vi "final_usrp_test.vi"() -> ()   [LabVIEW 2014]
uses:
  <vilib>/addons/Modulation/Analog/support/mod_Set Error Source.vi
  var_stop.vi
  <vilib>/addons/Modulation/Digital/Support/Common/Validators/mod_Generate Filter Coefficients Validate.vi
  <vilib>/addons/Modulation/Digital/General/subVIs/mod_Generate Filter Coefficients.vi
  <vilib>/measure/maspectr.llb/FFT Power Spectrum and PSD for 1 Chan (CDB).vi
  <vilib>/addons/Modulation/Digital/General/MT Apply Matched Filter (Generic).vi
  <vilib>/addons/Modulation/Digital/General/MT Align to Ideal Symbols (Generic).vi
  <instrlib>/niUSRP/niUSRP Fetch Rx Data (CDB Cluster).vi
  <instrlib>/niUSRP/niUSRP Write Tx Data (CDB Cluster).vi
  <vilib>/addons/Modulation/Digital/General/MT Apply Pulse Shaping Filter (Generic).vi
  <vilib>/addons/Modulation/niDMT.lvlib
  <vilib>/measure/NI_MAPro.lvlib
panel:
  out "energy detector  size":i32
  in  "frame buffer size":i32=20
  in  "Stop":bool
  out "Frames Per Second":u32
  in  "energy threshold":dbl=-33.0 format="%#_13g"
  out "elements in frame buffer 2":i32
  out "elements in frame buffer":i32
  out "valid frames":i32
  out "elements in send buffer":i32
  in  "packet size":i32=12800
  in  "Quality (0-1000)":i32=100 caption="Quality (750)"
  out "size(s) 4":i32
  out "frame num":u32
  out "length":i32[](array[numeric])
  out "start index":i32[](array[numeric])
  out "Numeric":i32
  out "size(s) 3":i32
  out "# elements in queue 2":i32
  out "size(s) 2":i32
  out "size(s)":i32[](array[numeric])
  out "image":T1(plugin-control)
  in  "Transmit power (db)":dbl
  out "found?":bool
  out "# elements in queue":i32
  out "valid?":bool
  in  "Gray code?":bool=TRUE
  in  "Modulation":enum16{"PSK", "QAM"}(ring)
  out "packet len":u32
  in  "filter length (symbols)":i32=8
  in  "filter parameter":dbl=0.5 format="%.2f"
  in  "pulse shaping filter (none)":T2(ring)=enum."Raised Cosine"
  in  "M-PSK (4)":i32=4 caption="M-ARY"
  in  "samples per symbol (16)":i32=4
  out "packet bits length":i32
  in  "number of samples":i64=40000
  out "RX coerced gain":dbl format="%#_6f"
  out "RX coerced carrier frequency":dbl=915000000.0 format="%#_6p"
  out "RX coerced IQ rate":dbl=4000000.0 format="%#_6p"
  in  "RX active antenna":string="RX2"
  in  "RX gain":dbl format="%#_6f"
  in  "RX device names":refnum<k15>="192.168.10.2"
  out "TX coerced gain":dbl format="%#_6f"
  out "TX coerced carrier frequency":dbl=915000000.0 format="%#_6p"
  out "coerced IQ rate":dbl=4000000.0 format="%#_6p"
  in  "TX device names":refnum<k15>="192.168.10.2"
  in  "TX gain":dbl format="%#_6f"
  in  "carrier frequency":dbl=915000000.0 format="%#_6p"
  in  "IQ rate":dbl=800000.0 format="%#_6p"
  in  "stop":bool
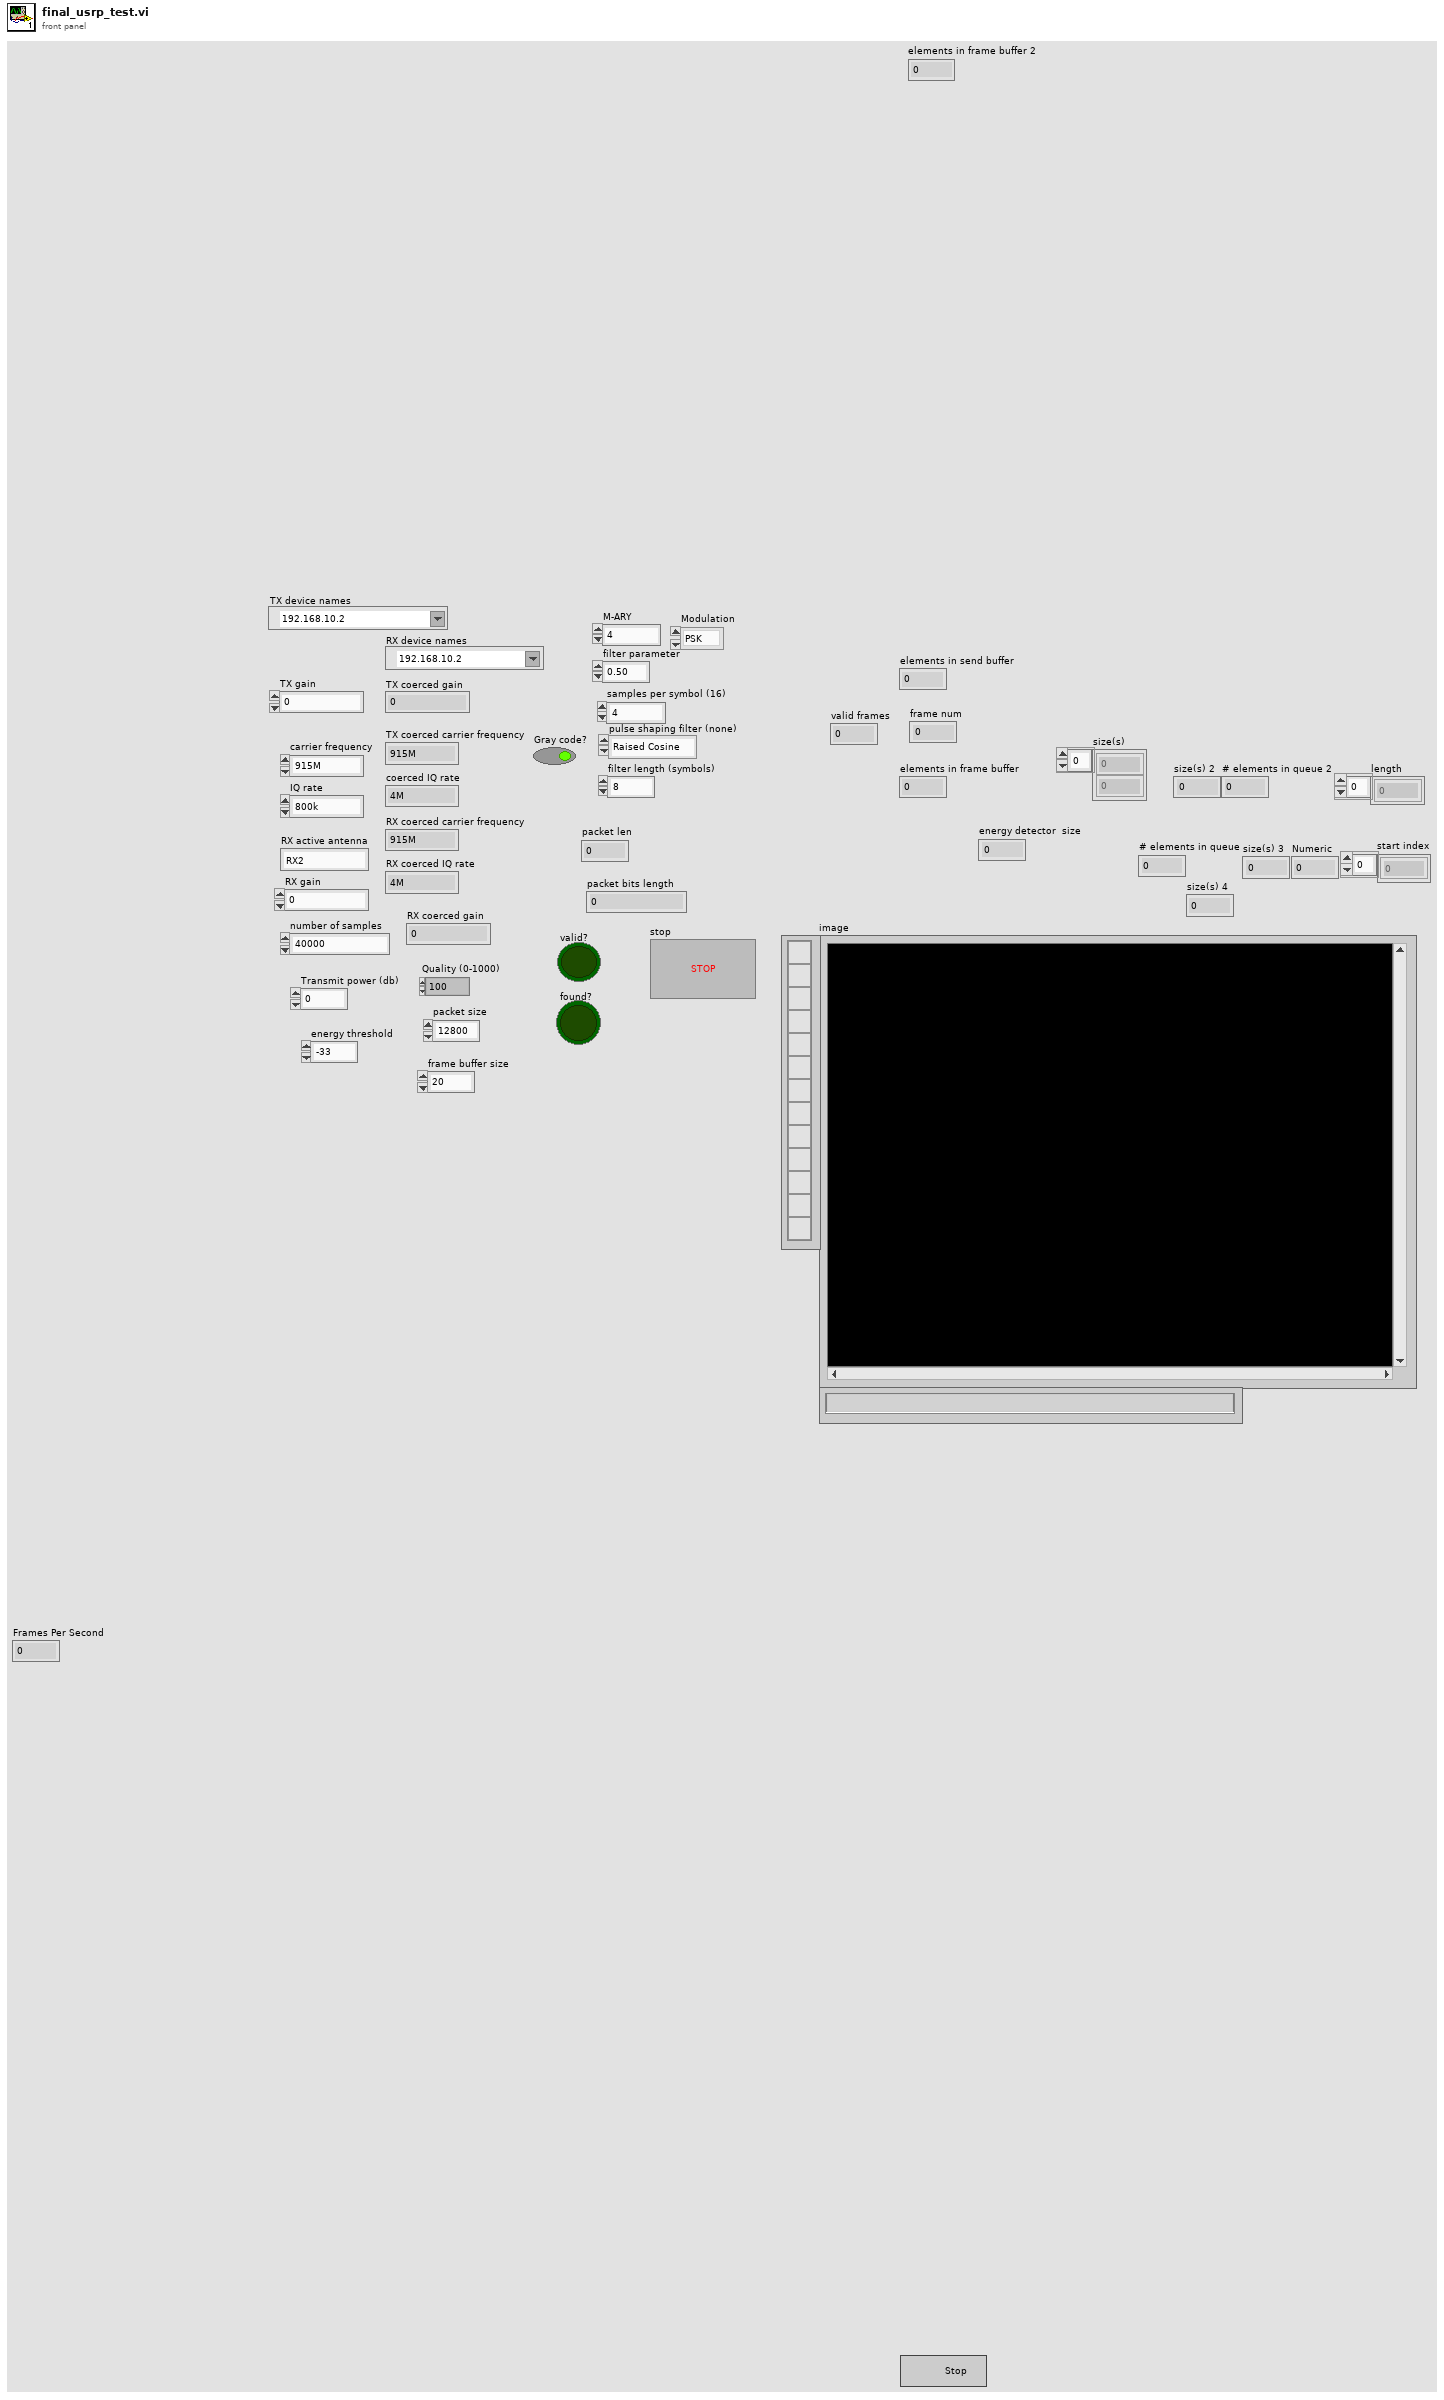
[diagram p1: front panel]
types:
  T1 = typedef "IMAQ Image.ctl" = refnum<image>
  T2 = enum16{"none", "Raised Cosine", "Root Raised Cos", "Gaussian"}
  T3 = enum16{"FSK", "PSK", "QAM", "MSK", "PAM", "ASK", "CPM"}
  T4 = cluster{"samples per symbol (16)":i32, "symbol map":cdb[], "index map":u32[]}
  T5 = cluster{"samples per symbol (16)":i32, "symbol map":cdb[], i32[]}
  T6 = typedef "IMAQ AVI2 Refnum.ctl" = refnum<k20>
  T7 = typedef "Image Type" = u32
  T8 = cluster{"Width":u32, "Height":u32, "Frames Per Second":u32, "Codec":string, "Has Data":bool}
  T9 = typedef "niAMT.lvlib/Complex Data Waveform.ctl" = cluster{"t0":dbl, "dt":dbl, "Y":cdb[]}
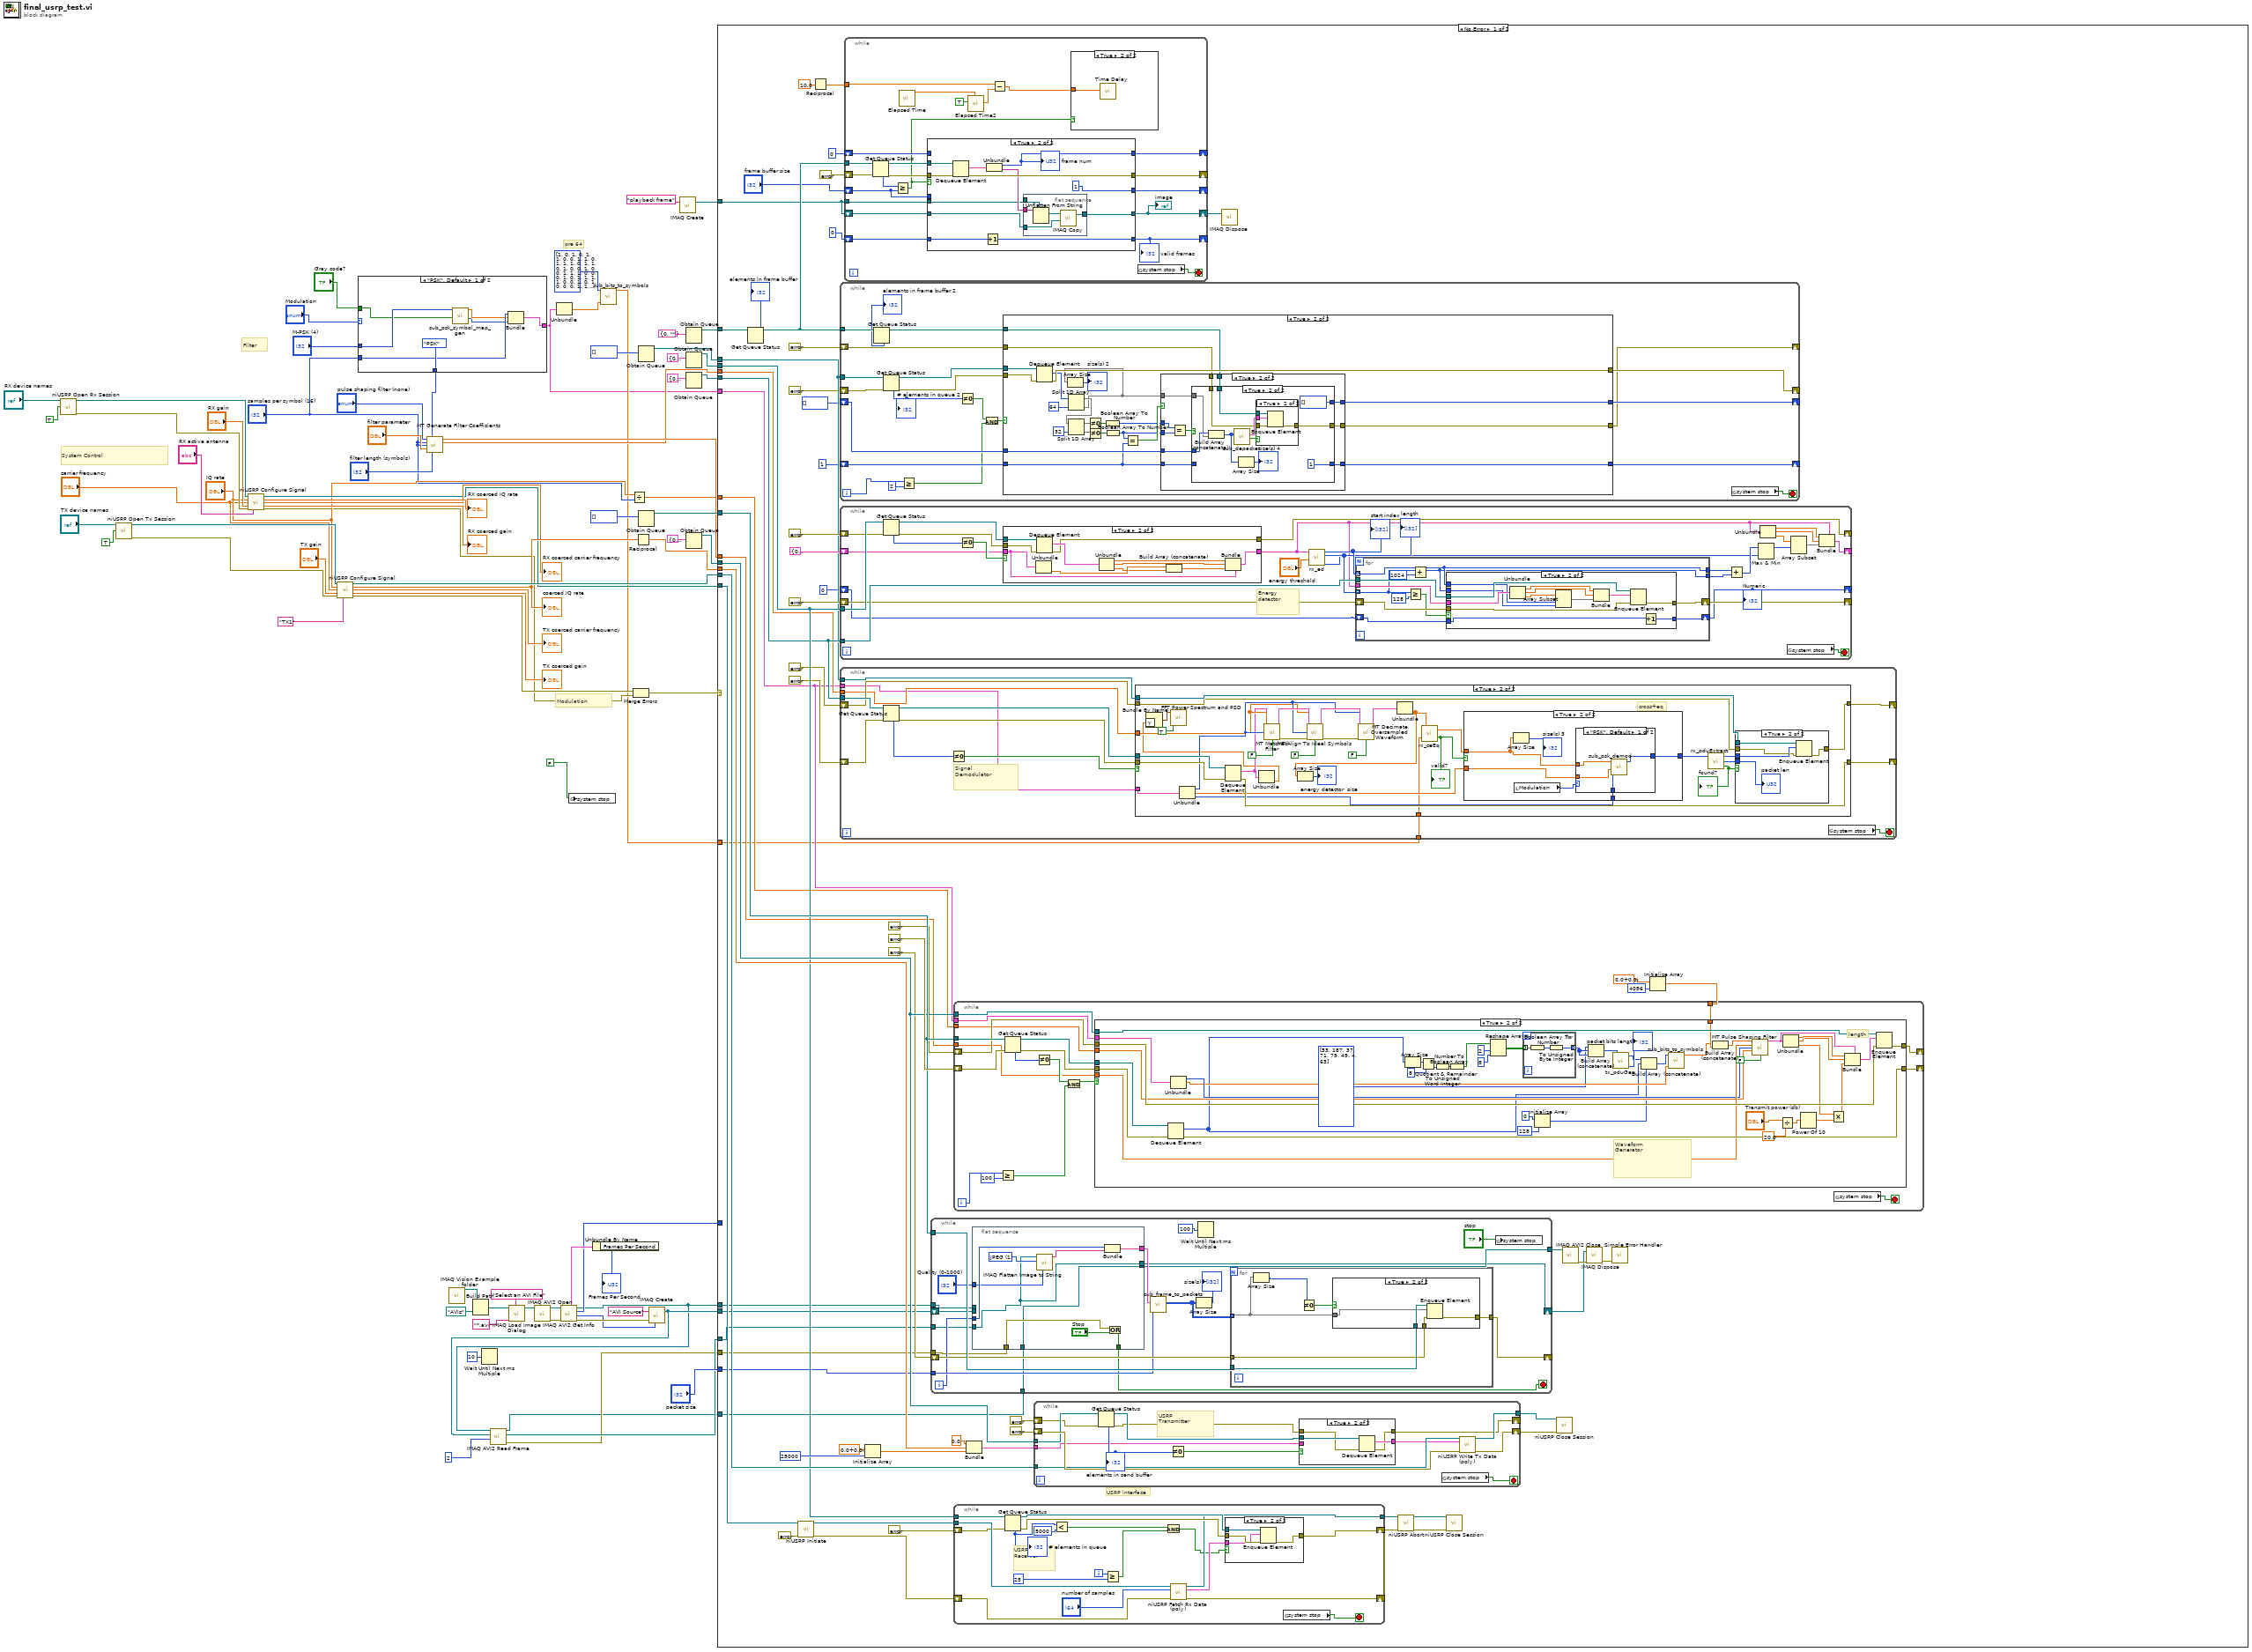
[diagram p0: block diagram]
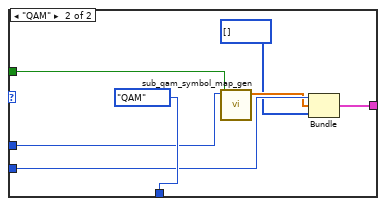
[diagram p2: hidden frame]
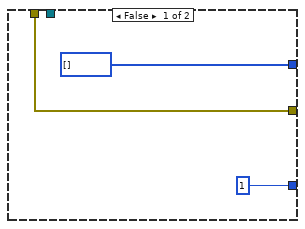
[diagram p7: hidden frame]
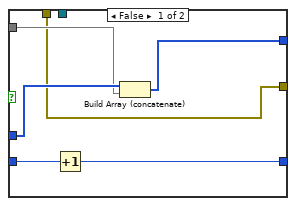
[diagram p8: hidden frame]
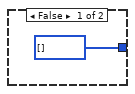
[diagram p11: hidden frame]
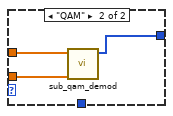
[diagram p12: hidden frame]
diagram:
  # "pre 64"
  # "Modulation"
  # "Filter"
  # "System Control"
  n1 = call <instrlib>:"niUSRP Open Rx Session.vi"("device names"="RX device names", "reset"=TRUE) -> ("session handle out"=w64:refnum<k15>, "error out"=w63:errorcluster)  [unwired: 12 in]
  n2 = call <instrlib>:"niUSRP Open Tx Session.vi"("device names"="TX device names", "reset"=TRUE) -> ("session handle out"=w77:refnum<k15>, "error out"=w76:errorcluster)  [unwired: 12 in]
  n3 = call <instrlib>:"niUSRP Configure Signal.vi"("session handle"=w64, "IQ rate"="IQ rate", "carrier frequency"="carrier frequency", "gain"="RX gain", "error in (no error)"=w63, "active antenna"="RX active antenna") -> ("session handle out"=w55:refnum<k15>, "coerced IQ rate"=→"RX coerced IQ rate":dbl, "coerced carrier frequency"=→"RX coerced carrier frequency":dbl, "coerced gain"=→"RX coerced gain":dbl, "error out"=w39:errorcluster)  [unwired: 5 in]
  n4 = call <instrlib>:"niUSRP Configure Signal.vi"("session handle"=w77, "IQ rate"="IQ rate", "carrier frequency"="carrier frequency", "gain"="TX gain", "error in (no error)"=w76, "active antenna"="TX1") -> ("session handle out"=w68:refnum<k15>, "coerced IQ rate"=w66:dbl, "coerced carrier frequency"=→"TX coerced carrier frequency":dbl, "coerced gain"=→"TX coerced gain":dbl, "error out"=w40:errorcluster)  [unwired: 5 in]
  "coerced IQ rate" <- w66
  n5 = case shown="\"PSK\", Default" "Modulation" {
    tunnel: [T3."PSK" ("modulation type") T3."QAM" ("modulation type")] -> w34
    tunnel: "M-PSK (4)" -> [w84 w90]
    tunnel: "Gray code?" -> [w83 w91]
    tunnel: "samples per symbol (16)" -> [w82 w89]
    tunnel: [w79 w86] -> w27
    frame "PSK", Default {
      n6 = call "sub_psk_symbol_map_gen.vi"("Gray code?"=w83, "M-PSK"=w84) -> ("index map"=w80:u32[], "symbol map"=w81:cdb[])  [unwired: 8 in]
      n7 = Bundle("samples per symbol (16)"=w82, "symbol map"=w81, "index map"=w80) -> (w79:T4)  [unwired: 1 in]
    }
    frame "QAM" {
      n8 = call "sub_qam_symbol_map_gen.vi"("Gray code?"=w91, "M-QAM"=w90) -> ("symbol map"=w88:cdb[])  [unwired: 9 in]
      n9 = Bundle("samples per symbol (16)"=w89, "symbol map"=w88, i32[] []) -> (w86:T5)  [unwired: 1 in]
    }
  }
  n10 = call <vilib>:"MT Generate Filter Coefficients.vi"("pulse shaping filter (none)"="pulse shaping filter (none)", "modulation type"=w34, "pulse shaping samples per symbol (16)"="samples per symbol (16)", "matched samples per symbol (16)"="samples per symbol (16)", "filter parameter"="filter parameter", "filter length (symbols)"="filter length (symbols)") -> ("pulse shaping filter coefficients"=w45:dbl[], "matched filter coefficients"=w43:dbl[])  [unwired: 7 in, 1 out]
  n11 = call "IMAQ Vision Example folder.vi"() -> ("Example Image Path"=w17:path)  [unwired: 11 in]
  n12 = Build Path(base path=w17, name or relative path=path "AVIs") -> (appended path=w14:path)
  n13 = Wait Until Next ms Multiple(millisecond multiple=u32 10) -> ()  [unwired: 1 out]
  n14 = call "IMAQ Load Image Dialog"("Prompt"="Select an AVI File" ("prompt"), "Pattern"="*.avi", "Start Path"=w14) -> ("Path"=w13:path)  [unwired: 6 in, 2 out]
  n15 = call "IMAQ AVI2 Open"("AVI File Path"=w13) -> ("error out"=w21:errorcluster, "AVI Refnum"=w20:T6)  [unwired: 2 in, 7 out]
  n16 = Unbundle(w27) -> ("symbol map"=w29:cdb[])  [unwired: 2 out]
  n17 = call "IMAQ AVI2 Get Info"("error in (no error)"=w21, "AVI Refnum"=w20) -> ("error out"=w19:errorcluster, "Image Type"=w18:T7, "Number of Frames"=w10:u32, "AVI Refnum (duplicate)"=w5:T6, "Frame Data"=w22:T8)  [unwired: 5 out]
  n18 = global write "var_stop.vi" "system stop"(FALSE) -> ()
  n19 = Unbundle By Name(w22) -> ("Frames Per Second"=→"Frames Per Second":u32)
  n20 = call "sub_bits_to_symbols.vi"("symbol map"=w29, "bits"=i16[] [1, 0, 1, 0, 1, 1, 0, 0, 1, 1, 0, 1, 1, 1, 0, 1, 1, 0, 1, 0, 0, 1, 0, 0, 1, 1, 1, 0, 0, 0, 1, 0, 1, 1, 1, 1, 0, 0, 1, 0, 1, 0, 0, 0, 1, 1, 0, 0, 0, 0, 1, 0, 0, 0, 0, 0, 1, 1, 1, 1, 1, 1, 0, 0] ("preamble(64) 2")) -> ("symbols"=w28:cdb[])  [unwired: 9 in]
  n21 = Divide(x="IQ rate", y="samples per symbol (16)") -> (x/y=w44:dbl)
  n22 = Merge Errors(w40, w39) -> (w38:errorcluster)
  n23 = Reciprocal(x=w66) -> (1/x=w65:dbl)
  n24 = Obtain Queue(element data type=i8[] [] ("output bit stream")) -> (queue out=w50:refnum<queue>)  [unwired: 4 in, 2 out]
  n25 = Obtain Queue(element data type=i16[] []) -> (queue out=w78:refnum<queue>)  [unwired: 4 in, 2 out]
  n26 = call "IMAQ Create"("Image Name"="AVI Source", "Image Type"=w18, "error in (no error)"=w19) -> ("New Image"=w6:T1)  [unwired: 1 in, 2 out]
  n27 = call "IMAQ AVI2 Read Frame"("Frame Number"=u32 2, "Image"=w6, "AVI Refnum"=w5) -> ("error out"=w2:errorcluster, "Image Out"=w3:T1, "AVI Refnum (duplicate)"=w1:T6)  [unwired: 1 in, 5 out]
  n28 = call "IMAQ Create"("Image Name"="playback frame") -> ("New Image"=w8:T1)  [unwired: 3 in, 2 out]
  n29 = Obtain Queue(element data type=cluster{u32, "string":string} {0, "string"=""} ("frame")) -> (queue out=w25:refnum<queue>)  [unwired: 4 in, 2 out]
  n30 = Obtain Queue(element data type=cluster{"t0":dbl, "dt":dbl, "Y":cdb[]} {"t0"=0.0, "dt"=0.0, "Y"=[]} ("data")) -> (queue out=w54:refnum<queue>)  [unwired: 4 in, 2 out]
  n31 = Obtain Queue(element data type=cluster{"t0":dbl, "dt":dbl, "Y":cdb[]} {"t0"=0.0, "dt"=0.0, "Y"=[]} ("data")) -> (queue out=w51:refnum<queue>)  [unwired: 4 in, 2 out]
  n32 = Obtain Queue(element data type=cluster{"t0":dbl, "dt":dbl, "Y":cdb[]} {"t0"=0.0, "dt"=1.0, "Y"=[]} ("data")) -> (queue out=w69:refnum<queue>)  [unwired: 4 in, 2 out]
  n33 = case shown="No Error" w38 {
    tunnel: w78 -> [w158 _]
    tunnel: w69 -> [w153 _]
    tunnel: w68 -> [w154 _]
    tunnel: w65 -> [w147 _]
    tunnel: w55 -> [w142 _]
    tunnel: w54 -> [w136 _]
    tunnel: w51 -> [w132 _]
    tunnel: w50 -> [w130 _]
    tunnel: w27 -> [w124 _]
    tunnel: w45 -> [w127 _]
    tunnel: w44 -> [w126 _]
    tunnel: w43 -> [w125 _]
    tunnel: w28 -> [w118 _]
    tunnel: w25 -> [w114 _]
    tunnel: "packet size" -> [w108 _]
    tunnel: w10 -> [_ _]
    tunnel: w5 -> [w103 _]
    tunnel: w6 -> [w102 _]
    tunnel: w8 -> [w96 _]
    tunnel: w3 -> [w95 _]
    tunnel: w2 -> [w94 _]
    tunnel: w1 -> [w93 _]
    frame No Error {
      # "USRP interface"
      n34 = Get Queue Status(queue=w114) -> (queue out=w106:refnum<queue>, # elements in queue=→"elements in frame buffer":i32)  [unwired: 2 in, 6 out]
      n35 = call <instrlib>:"niUSRP Initiate.vi"("session handle"=w142, "error in (no error)"=errorcluster {"status"=FALSE, "code"=0, "source"=""}) -> ("session handle out"=w141:refnum<k15>, "error out"=w140:errorcluster)  [unwired: 12 in]
      n36 = Reciprocal(x=10.0) -> (1/x=w109:dbl)
      n37 = while {
        tunnel: w130 -> [w265]
        shift-right: [w258] -> _
        shift-left: errorcluster {"status"=FALSE, "code"=0, "source"=""} ("error out") -> [w264]
        shift-right: [w256] -> _
        shift-left: u32 1 -> [w257]
        shift-right: [w255] -> _
        shift-left: i8[] [] ("second subarray") -> [w254]
        tunnel: w106 -> [w253]
        shift-right: [w251] -> _
        shift-left: errorcluster {"status"=FALSE, "code"=0, "source"=""} ("error out") -> [w252]
        i -> [w249]
        stop <- w263 stop-if-true
        n38 = Get Queue Status(queue=w253) -> (queue out=w246:refnum<queue>, # elements in queue=→"elements in frame buffer 2":i32)  [unwired: 2 in, 6 out]
        n39 = Get Queue Status(queue=w265, error in (no error)=w264) -> (queue out=w260:refnum<queue>, error out=w259:errorcluster, # elements in queue=w262:i32)  [unwired: 1 in, 5 out]
        "# elements in queue 2" <- w262
        n40 = Greater Or Equal?(x=w249, y=2) -> (x >= y?=w248:bool)
        n41 = Not Equal To 0?(x=w262) -> (x != 0?=w261:bool)
        n42 = And(x=w261, y=w248) -> (x .and. y?=w247:bool)
        n43 = case shown="True" w247 {
          tunnel: w260 -> [_ w292]
          tunnel: w259 -> [w269 w291]
          tunnel: [w269 w290] -> w258
          tunnel: w257 -> [w268 w276]
          tunnel: [w268 w277] -> w256
          tunnel: [w266 w281] -> w255
          tunnel: w254 -> [w266 w278]
          tunnel: w246 -> [_ w275]
          tunnel: w252 -> [w267 w274]
          tunnel: [w267 w273] -> w251
          frame False {
          }
          frame True {
            n44 = Dequeue Element(queue=w292, error in (no error)=w291) -> (element=w272:i8[], error out=w290:errorcluster)  [unwired: 1 in, 2 out]
            n45 = Split 1D Array(array=w272, index=64) -> (first subarray=w283:i8[], second subarray=w270:i8[])
            n46 = Array Size(array=w270) -> (size(s)=→"size(s) 2":i32)
            n47 = Split 1D Array(array=w283, index=32) -> (first subarray=w286:i8[], second subarray=w287:i8[])
            n48 = Not Equal To 0?(x=w286) -> (x != 0?=w285:bool[])
            n49 = Not Equal To 0?(x=w287) -> (x != 0?=w284:bool[])
            n50 = Boolean Array To Number(Boolean array=w285) -> (number=w280:u32)
            n51 = Boolean Array To Number(Boolean array=w284) -> (number=w279:u32)
            n52 = Equal?(x=w279, y=w276) -> (x = y?=w282:bool)
            n53 = case shown="True" w282 {
              tunnel: [i8[] [] ("second subarray") w303] -> w281
              tunnel: w280 -> [_ w306]
              tunnel: w279 -> [_ w305]
              tunnel: w278 -> [_ w302]
              tunnel: w270 -> [_ w301]
              tunnel: [u32 1 w300] -> w277
              tunnel: w276 -> [_ w299]
              tunnel: w275 -> [_ w298]
              tunnel: w274 -> [w293 w297]
              tunnel: [w293 w296] -> w273
              frame False {
              }
              frame True {
                n54 = Equal?(x=w306, y=w305) -> (x = y?=w304:bool)
                n55 = case shown="True" w304 {
                  tunnel: [w310 i8[] [] ("second subarray")] -> w303
                  tunnel: w302 -> [w312 w321]
                  tunnel: w301 -> [w311 w320]
                  tunnel: [w308 u32 1] -> w300
                  tunnel: w299 -> [w309 _]
                  tunnel: w298 -> [_ w319]
                  tunnel: w297 -> [w307 w317]
                  tunnel: [w307 w316] -> w296
                  frame False {
                    n56 = Increment(x=w309) -> (x+1=w308:u32)
                    n57 = Build Array (concatenate)(w312, w311) -> (w310:i8[])
                  }
                  frame True {
                    n58 = Build Array (concatenate)(w321, w320) -> (w315:i8[])
                    n59 = call "sub_depacket.vi"("bitstream"=w315) -> ("CRC valid"=w313:bool, "frame"=w318:cluster{u32, "string":string})  [unwired: 9 in]
                    n60 = Array Size(array=w315) -> (size(s)=→"size(s) 4":i32)
                    n61 = case shown="True" w313 {
                      tunnel: w319 -> [_ w328]
                      tunnel: w318 -> [_ w327]
                      tunnel: w317 -> [w324 w326]
                      tunnel: [w324 w325] -> w316
                      frame False {
                      }
                      frame True {
                        n62 = Enqueue Element(queue=w328, element=w327, error in (no error)=w326) -> (error out=w325:errorcluster)  [unwired: 1 in, 2 out]
                      }
                    }
                  }
                }
              }
            }
          }
        }
        n63 = global read "var_stop.vi" "system stop"() -> (w263:bool)
      }
      n64 = while {
        tunnel: w136 -> [w424]
        shift-right: [w417] -> _
        shift-left: errorcluster {"status"=FALSE, "code"=0, "source"=""} ("error out") -> [w423]
        shift-right: [w403] -> _
        shift-left: cluster{"t0":dbl, "dt":dbl, "Y":cdb[]} {"t0"=0.0, "dt"=0.0, "Y"=[]} ("data") -> [w418]
        tunnel: w132 -> [w416]
        shift-right: [w415] -> _
        shift-left: errorcluster {"status"=FALSE, "code"=0, "source"=""} ("error out") -> [w414]
        shift-right: [w398] -> _
        shift-left: 0 -> [w399]
        stop <- w413 stop-if-true
        # "Energy\ndetector"
        n65 = Get Queue Status(queue=w424, error in (no error)=w423) -> (queue out=w419:refnum<queue>, error out=w420:errorcluster, # elements in queue=w422:i32)  [unwired: 1 in, 5 out]
        n66 = Not Equal To 0?(x=w422) -> (x != 0?=w421:bool)
        n67 = case shown="True" w421 {
          tunnel: w420 -> [w453 w464]
          tunnel: w419 -> [_ w463]
          tunnel: w418 -> [w452 w458]
          tunnel: [w453 w455] -> w417
          tunnel: [w452 w454] -> w410
          frame False {
          }
          frame True {
            n68 = Unbundle(w458) -> ("Y"=w461:cdb[])  [unwired: 2 out]
            n69 = Dequeue Element(queue=w463, error in (no error)=w464) -> (element=w462:cluster{"t0":dbl, "dt":dbl, "Y":cdb[]}, error out=w455:errorcluster)  [unwired: 1 in, 2 out]
            n70 = Unbundle(w462) -> ("t0"=w457:dbl, "dt"=w456:dbl, "Y"=w460:cdb[])
            n71 = Build Array (concatenate)(w461, w460) -> (w459:cdb[])
            n72 = Bundle(cluster=w458, "t0"=w457, "dt"=w456, "Y"=w459) -> (w454:cluster{"t0":dbl, "dt":dbl, "Y":cdb[]})
          }
        }
        n73 = call "rx_ed.vi"("energy threshold"="energy threshold", "Wavefrom"=w410) -> ("first pulse"=w400:i32, "length"=w411:i32[], "start index"=w412:i32[])  [unwired: 7 in]
        "start index" <- w412
        "length" <- w411
        n74 = for {
          tunnel: w416 -> [w436]
          tunnel: w410 -> [w433]
          shift-right: [w435] -> w415
          shift-left: w414 -> [w434]
          tunnel: w412 -> [w432] mode=indexing
          tunnel: w411 -> [w431] mode=indexing
          tunnel: [w432] -> w406
          tunnel: [w426] -> w405
          shift-right: [w427] -> w398
          shift-left: w399 -> [w428]
          n75 = Greater Or Equal?(x=w431, y=128) -> (x >= y?=w429:bool)
          n76 = Add(x=w431, y=1024) -> (x+y=w426:i32)
          n77 = case shown="True" w429 {
            tunnel: w436 -> [_ w451]
            tunnel: [w438 w450] -> w435
            tunnel: w434 -> [w438 w449]
            tunnel: w433 -> [_ w448]
            tunnel: w432 -> [_ w442]
            tunnel: w426 -> [_ w441]
            tunnel: w428 -> [w437 w440]
            tunnel: [w437 w439] -> w427
            frame False {
            }
            frame True {
              n78 = Unbundle(w448) -> ("t0"=w446:dbl, "dt"=w447:dbl, "Y"=w444:cdb[])
              n79 = Array Subset(array=w444, index=w442, length=w441) -> (w443:cdb[])
              n80 = Bundle("t0"=w446, "dt"=w447, w443) -> (w445:cluster{"t0":dbl, "dt":dbl, cdb[]})  [unwired: 1 in]
              n81 = Enqueue Element(queue=w451, element=w445, error in (no error)=w449) -> (error out=w450:errorcluster)  [unwired: 1 in, 2 out]
              n82 = Increment(x=w440) -> (x+1=w439:i32)
            }
          }
        }
        "Numeric" <- w398
        n83 = Add(x=w406, y=w405) -> (x+y=w402:i32)
        n84 = Max & Min(x=w402, y=w400) -> (max(x,y)=w401:i32)  [unwired: 1 out]
        n85 = Unbundle(w410) -> ("t0"=w409:dbl, "dt"=w408:dbl, "Y"=w407:cdb[])
        n86 = global read "var_stop.vi" "system stop"() -> (w413:bool)
        n87 = Array Subset(array=w407, index=w401) -> (w404:cdb[])  [unwired: 1 in]
        n88 = Bundle(cluster=w410, "t0"=w409, "dt"=w408, "Y"=w404) -> (w403:cluster{"t0":dbl, "dt":dbl, "Y":cdb[]})
      }
      n89 = while {
        tunnel: w132 -> [w342]
        shift-right: [w336] -> _
        shift-left: errorcluster {"status"=FALSE, "code"=0, "source"=""} ("error out") -> [w341]
        tunnel: w130 -> [w335]
        shift-right: [w334] -> _
        shift-left: errorcluster {"status"=FALSE, "code"=0, "source"=""} ("error out") -> [w333]
        tunnel: w125 -> [w331]
        tunnel: w124 -> [w330]
        tunnel: w118 -> [w329]
        stop <- w332 stop-if-true
        # "Signal \nDemodulator"
        n90 = Get Queue Status(queue=w342, error in (no error)=w341) -> (queue out=w338:refnum<queue>, error out=w337:errorcluster, # elements in queue=w340:i32)  [unwired: 1 in, 5 out]
        n91 = Not Equal To 0?(x=w340) -> (x != 0?=w339:bool)
        n92 = case shown="True" w339 {
          tunnel: w338 -> [_ w375]
          tunnel: w337 -> [w344 w376]
          tunnel: [w344 w374] -> w336
          tunnel: w335 -> [_ w365]
          tunnel: [w343 w364] -> w334
          tunnel: w333 -> [w343 w363]
          tunnel: w331 -> [_ w352]
          tunnel: w330 -> [_ w356]
          tunnel: w329 -> [_ w349]
          frame False {
          }
          frame True {
            # "cross+eq"
            n93 = Unbundle(w356) -> ("samples per symbol (16)"=w355:i32, "symbol map"=w354:cdb[], "index map"=w353:u32[])
            n94 = Dequeue Element(queue=w375, error in (no error)=w376) -> (element=w348:cluster{"t0":dbl, "dt":dbl, "Y":cdb[]}, error out=w374:errorcluster)  [unwired: 1 in, 2 out]
            n95 = Unbundle(w348) -> ("Y"=w347:cdb[])  [unwired: 2 out]
            n96 = Bundle By Name("Y"=w347) -> (w351:waveform(cdb))  [unwired: 1 in]
            n97 = call-poly <vilib>:"FFT Power Spectrum and PSD.vi"("dB On (F)"=TRUE, "time signal"=w351) -> ()  [unwired: 6 in, 4 out]
            n98 = call-poly <vilib>:"MT Matched Filter.vi"("input complex waveform"=w348, "matched filter coefficients"=w352, "samples per symbol (16)"=w355, "reset? (T)"=FALSE) -> ("output complex waveform"=w373:T9, "error out"=w372:errorcluster)  [unwired: 10 in]
            n99 = call-poly <vilib>:"MT Align To Ideal Symbols.vi"("input complex waveform"=w373, "matched filter coefficients"=w352, "samples per symbol (16)"=w355, "error in (no error)"=w372, "reset? (T)"=FALSE) -> ("output complex waveform"=w370:T9, "error out"=w371:errorcluster)  [unwired: 8 in, 1 out]
            n100 = call <vilib>:"MT Decimate Oversampled Waveform.vi"("input complex waveform"=w370, "decimation factor"=w355, "error in (no error)"=w371, "reset? (T)"=FALSE) -> ("output complex waveform"=w369:T9)  [unwired: 10 in, 1 out]
            n101 = Unbundle(w369) -> ("Y"=w345:cdb[])  [unwired: 2 out]
            n102 = Array Size(array=w345) -> (size(s)=→"energy detector  size":i32)
            n103 = call "rx_ceEq.vi"("preamble"=w349, "symbols"=w345) -> ("valid?"=w361:bool, "eq symbols"=w362:cdb[])
            "valid?" <- w361
            n104 = case shown="True" w361 {
              tunnel: [i8[] [] ("output bit stream") w381] -> w368
              tunnel: w354 -> [_ w382]
              tunnel: w362 -> [_ w379]
              tunnel: w353 -> [_ w380]
              frame False {
              }
              frame True {
                n105 = Array Size(array=w379) -> (size(s)=→"size(s) 3":i32)
                n106 = local read "Modulation"() -> (w383:enum16{"PSK", "QAM"})
                n107 = case shown="\"PSK\", Default" w383 {
                  tunnel: w379 -> [w387 w390]
                  tunnel: w382 -> [w386 w389]
                  tunnel: [w384 w388] -> w381
                  tunnel: w380 -> [w385 _]
                  frame "PSK", Default {
                    n108 = call "sub_psk_demod.vi"("index map"=w385, "symbol map"=w386, "symbol"=w387) -> ("bitstream"=w384:i16[])  [unwired: 8 in]
                  }
                  frame "QAM" {
                    n109 = call "sub_qam_demod.vi"("symbol map"=w389, "symbol"=w390) -> ("bitstream"=w388:i16[])  [unwired: 9 in]
                  }
                }
              }
            }
            n110 = call "rx_pduExtract.vi"("output bit stream"=w368) -> ("found?"=w367:bool, "packet len"=w360:u32, "ppdu"=w366:i8[])  [unwired: 2 in]
            "found?" <- w367
            n111 = case shown="True" w367 {
              tunnel: w366 -> [_ w394]
              tunnel: w365 -> [_ w396]
              tunnel: [w391 w395] -> w364
              tunnel: w363 -> [w391 w392]
              tunnel: w360 -> [_ w393]
              frame False {
              }
              frame True {
                n112 = Enqueue Element(queue=w396, element=w394, error in (no error)=w392) -> (error out=w395:errorcluster)  [unwired: 1 in, 2 out]
                "packet len" <- w393
              }
            }
          }
        }
        n113 = global read "var_stop.vi" "system stop"() -> (w332:bool)
      }
      n114 = while {
        tunnel: w106 -> [w221]
        shift-right: [w217] -> _
        shift-left: errorcluster {"status"=FALSE, "code"=0, "source"=""} ("error out") -> [w220]
        shift-right: [w214] -> _
        shift-left: 0 -> [w213]
        tunnel: w109 -> [w209]
        shift-right: [w210] -> _
        shift-left: 0 -> [w211]
        shift-right: [w205] -> _
        shift-left: "frame buffer size" -> [w204]
        shift-right: [w201] -> w97
        shift-left: w96 -> [w202]
        tunnel: w96 -> [w200]
        stop <- w216 stop-if-true
        n115 = Get Queue Status(queue=w221, error in (no error)=w220) -> (queue out=w219:refnum<queue>, error out=w218:errorcluster, # elements in queue=w206:i32)  [unwired: 1 in, 5 out]
        n116 = Greater Or Equal?(x=w206, y=w204) -> (x >= y?=w203:bool)
        n117 = call "Elapsed Time"() -> ("Present (s)"=w208:dbl)  [unwired: 12 in, 7 out]
        n118 = case shown="True" w203 {
          tunnel: w219 -> [_ w239]
          tunnel: w218 -> [w227 w238]
          tunnel: [w227 w236] -> w217
          tunnel: [w226 w234] -> w214
          tunnel: w213 -> [w226 _]
          tunnel: w211 -> [w225 w233]
          tunnel: [w225 w232] -> w210
          tunnel: [w224 1] -> w205
          tunnel: w204 -> [w224 _]
          tunnel: [w223 w229] -> w201
          tunnel: w202 -> [w223 w228]
          tunnel: w200 -> [_ w230]
          frame False {
          }
          frame True {
            n119 = Dequeue Element(queue=w239, error in (no error)=w238) -> (element=w237:cluster{u32, "string":string}, error out=w236:errorcluster)  [unwired: 1 in, 2 out]
            n120 = Increment(x=w233) -> (x+1=w232:i32)
            n121 = Unbundle(w237) -> (w234:u32, "string"=w235:string)
            "frame num" <- w234
            n122 = flat-sequence {
              tunnel: w235 -> [w244]
              tunnel: w230 -> [w243]
              tunnel: [w241] -> w229
              tunnel: w228 -> [w240]
              frame #0 {
                n123 = Unflatten From String(type=w243, binary string=w244) -> (value=w242:T1)  [unwired: 3 in, 2 out]
                n124 = call "IMAQ Copy"("Image Dst"=w240, "Image Src"=w242) -> ("Image Dst Out"=w241:T1)  [unwired: 4 in, 1 out]
              }
            }
          }
        }
        "valid frames" <- w210
        "image" <- w201
        n125 = call "Elapsed Time2"("Reset"=TRUE, "Set Start Time (s)"=w208) -> ("Elapsed Time (s)"=w212:dbl)  [unwired: 10 in, 7 out]
        n126 = Subtract(x=w209, y=w212) -> (x-y=w207:dbl)
        n127 = case shown="True" w203 {
          tunnel: w207 -> [_ w222]
          frame False {
          }
          frame True {
            n128 = call "Time Delay"("Delay Time (s)"=w222) -> ()  [unwired: 10 in, 1 out]
          }
        }
        n129 = global read "var_stop.vi" "system stop"() -> (w216:bool)
      }
      n130 = Initialize Array(cdb 0.0+0.0i, 25000 ("dimension size")) -> (w148:cdb[])
      n131 = while {
        tunnel: w158 -> [w177]
        shift-right: [w175] -> _
        shift-left: errorcluster {"status"=FALSE, "code"=0, "source"=""} ("error out") -> [w176]
        tunnel: w108 -> [w171]
        tunnel: w103 -> [w167]
        tunnel: [w166] -> w99
        shift-right: [w165] -> w98
        shift-left: w102 -> [w170]
        tunnel: w95 -> [w162]
        tunnel: w94 -> [w161]
        tunnel: w93 -> [w160]
        i -> [w169]
        stop <- w164 stop-if-true
        n132 = flat-sequence {
          tunnel: w170 -> [_]
          tunnel: w169 -> [w185]
          tunnel: [w184] -> w168
          tunnel: w167 -> [_]
          tunnel: [w179] -> w166
          tunnel: [w180] -> w165
          tunnel: [w183] -> w164
          tunnel: "Quality (0-1000)" -> [w182]
          tunnel: w162 -> [w180]
          tunnel: w161 -> [w181]
          tunnel: w160 -> [w179]
          frame #0 {
            w187 = 1 items=["None", "JPEG", "PACKED BINARY"] ("Compression (None)")
            n133 = call "IMAQ Flatten Image to String"("Quality (750)"=w182, "Compression (None)"=w187, "Image"=w180) -> ("Data String"=w186:string)  [unwired: 7 in, 1 out]
            n134 = Bundle(w185, "Data String"=w186) -> (w184:cluster{i32, "Data String":string})  [unwired: 1 in]
            n135 = Or(x=w181, y="Stop") -> (x .or. y?=w183:bool)
          }
        }
        n136 = call "sub_frame_to_packets.vi"("packet size"=w171, "Cluster"=w168) -> ("packets"=w174:i16[][])  [unwired: 9 in]
        n137 = Array Size(array=w174) -> (size(s)=→"size(s)":i32[])
        n138 = Wait Until Next ms Multiple(millisecond multiple=u32 100) -> ()  [unwired: 1 out]
        n139 = for {
          tunnel: w177 -> [w194]
          tunnel: w176 -> [w193]
          tunnel: [w192] -> w175
          tunnel: w174 -> [w189] mode=indexing
          n140 = Array Size(array=w189) -> (size(s)=w190:i32)
          n141 = Not Equal To 0?(x=w190) -> (x != 0?=w191:bool)
          n142 = case shown="True" w191 {
            tunnel: w189 -> [_ w196]
            tunnel: w194 -> [_ w199]
            tunnel: w193 -> [w195 w198]
            tunnel: [w195 w197] -> w192
            frame False {
            }
            frame True {
              n143 = Enqueue Element(queue=w199, element=w196, error in (no error)=w198) -> (error out=w197:errorcluster)  [unwired: 1 in, 2 out]
            }
          }
        }
        n144 = global write "var_stop.vi" "system stop"("stop") -> ()
      }
      n145 = while {
        tunnel: w141 -> [w483]
        shift-right: [w472] -> w137
        shift-left: w140 -> [w482]
        tunnel: w136 -> [w480]
        shift-right: [w474] -> _
        shift-left: errorcluster {"status"=FALSE, "code"=0, "source"=""} ("error out") -> [w479]
        tunnel: [w473] -> w138
        i -> [w470]
        stop <- w471 stop-if-true
        # "USRP\nReceiver"
        n146 = Get Queue Status(queue=w480, error in (no error)=w479) -> (queue out=w476:refnum<queue>, error out=w475:errorcluster, # elements in queue=w478:i32)  [unwired: 1 in, 5 out]
        "# elements in queue" <- w478
        n147 = Less?(x=w478, y=5000) -> (x < y?=w468:bool)
        n148 = Greater Or Equal?(x=w470, y=25) -> (x >= y?=w467:bool)
        n149 = And(x=w468, y=w467) -> (x .and. y?=w465:bool)
        n150 = call-poly <instrlib>:"niUSRP Fetch Rx Data (poly).vi"("session handle"=w483, "number of samples"="number of samples", "error in (no error)"=w482) -> ("session handle out"=w473:refnum<k15>, "data"=w466:cluster{"t0":dbl, "dt":dbl, "Y":cdb[]}, "error out"=w472:errorcluster)  [unwired: 9 in, 1 out]
        n151 = case shown="True" w465 {
          tunnel: w476 -> [_ w488]
          tunnel: w475 -> [w484 w487]
          tunnel: [w484 w486] -> w474
          tunnel: w466 -> [_ w485]
          frame False {
          }
          frame True {
            n152 = Enqueue Element(queue=w488, element=w485, error in (no error)=w487) -> (error out=w486:errorcluster)  [unwired: 1 in, 2 out]
          }
        }
        n153 = global read "var_stop.vi" "system stop"() -> (w471:bool)
      }
      n154 = Bundle(0.0, w147, w148) -> (w145:cluster{dbl, dbl, cdb[]})  [unwired: 1 in]
      n155 = while {
        shift-right: [w498] -> w157
        shift-left: errorcluster {"status"=FALSE, "code"=0, "source"=""} ("error out") -> [w496]
        tunnel: [w497] -> w156
        tunnel: w154 -> [w495]
        tunnel: w153 -> [w493]
        shift-right: [w491] -> _
        shift-left: errorcluster {"status"=FALSE, "code"=0, "source"=""} ("error out") -> [w492]
        tunnel: w145 -> [w490]
        stop <- w489 stop-if-true
        # "USRP\nTransmitter"
        n156 = Get Queue Status(queue=w493, error in (no error)=w492) -> (queue out=w500:refnum<queue>, error out=w499:errorcluster, # elements in queue=w502:i32)  [unwired: 1 in, 5 out]
        "elements in send buffer" <- w502
        n157 = Not Equal To 0?(x=w502) -> (x != 0?=w501:bool)
        n158 = case shown="True" w501 {
          tunnel: w500 -> [_ w508]
          tunnel: w499 -> [w503 w507]
          tunnel: [w504 w506] -> w494
          tunnel: [w503 w505] -> w491
          tunnel: w490 -> [w504 _]
          frame False {
          }
          frame True {
            n159 = Dequeue Element(queue=w508, error in (no error)=w507) -> (element=w506:cluster{"t0":dbl, "dt":dbl, "Y":cdb[]}, error out=w505:errorcluster)  [unwired: 1 in, 2 out]
          }
        }
        n160 = global read "var_stop.vi" "system stop"() -> (w489:bool)
        n161 = call-poly <instrlib>:"niUSRP Write Tx Data (poly).vi"("session handle"=w495, "data"=w494, "error in (no error)"=w496) -> ("session handle out"=w497:refnum<k15>, "error out"=w498:errorcluster)  [unwired: 11 in]
      }
      n162 = call "IMAQ Dispose"("Image"=w97) -> ()  [unwired: 2 in, 4 out]
      n163 = call <instrlib>:"niUSRP Abort.vi"("session handle"=w138, "error in (no error)"=w137) -> ("session handle out"=w144:refnum<k15>, "error out"=w143:errorcluster)  [unwired: 12 in]
      n164 = call <instrlib>:"niUSRP Close Session.vi"("session handle"=w144, "error in (no error)"=w143) -> ()  [unwired: 13 in, 1 out]
      n165 = call <instrlib>:"niUSRP Close Session.vi"("session handle"=w156, "error in (no error)"=w157) -> ()  [unwired: 13 in, 1 out]
      n166 = call "IMAQ AVI2 Close"("AVI Refnum"=w99) -> ("error out"=w100:errorcluster)  [unwired: 1 in, 9 out]
      n167 = call "IMAQ Dispose"("Image"=w98, "error in (no error)"=w100) -> ("error out"=w101:errorcluster)  [unwired: 1 in, 3 out]
      n168 = call <vilib>:"Simple Error Handler.vi"("error in (no error)"=w101) -> ()  [unwired: 1 in, 8 out]
      n169 = Initialize Array(cdb 0.0+0.0i, 4096 ("dimension size")) -> (w119:cdb[])
      n170 = while {
        tunnel: w158 -> [w524]
        shift-right: [w521] -> _
        shift-left: errorcluster {"status"=FALSE, "code"=0, "source"=""} ("error out") -> [w527]
        tunnel: w153 -> [w520]
        shift-right: [w519] -> _
        shift-left: errorcluster {"status"=FALSE, "code"=0, "source"=""} ("error out") -> [w518]
        tunnel: w124 -> [w516]
        tunnel: w127 -> [w515]
        tunnel: w126 -> [w514]
        tunnel: w119 -> [w513]
        i -> [w512]
        stop <- w517 stop-if-true
        n171 = Greater Or Equal?(x=w512, y=100) -> (x >= y?=w509:bool)
        n172 = Get Queue Status(queue=w524, error in (no error)=w527) -> (queue out=w522:refnum<queue>, error out=w523:errorcluster, # elements in queue=w526:i32)  [unwired: 1 in, 5 out]
        n173 = Not Equal To 0?(x=w526) -> (x != 0?=w525:bool)
        n174 = And(x=w525, y=w509) -> (x .and. y?=w510:bool)
        n175 = case shown="True" w510 {
          tunnel: w523 -> [w529 w572]
          tunnel: w522 -> [_ w571]
          tunnel: [w529 w570] -> w521
          tunnel: w520 -> [_ w565]
          tunnel: [w528 w564] -> w519
          tunnel: w518 -> [w528 w563]
          tunnel: w516 -> [_ w560]
          tunnel: w515 -> [_ w559]
          tunnel: w514 -> [_ w558]
          tunnel: w513 -> [_ w548]
          frame False {
          }
          frame True {
            # "length"
            # "Waveform \nGenerator"
            n176 = Dequeue Element(queue=w571, error in (no error)=w572) -> (element=w532:i16[], error out=w570:errorcluster)  [unwired: 1 in, 2 out]
            n177 = Unbundle(w560) -> ("samples per symbol (16)"=w554:i32, "symbol map"=w547:cdb[])  [unwired: 1 out]
            n178 = Array Size(array=w532) -> (size(s)=w556:i32)
            n179 = Quotient & Remainder(x=w556, y=8) -> (floor(x/y)=w536:i32)  [unwired: 1 out]
            n180 = To Unsigned Word Integer(number=w536) -> (unsigned 16bit integer=w555:u16)
            n181 = Number To Boolean Array(number=w555) -> (Boolean array=w569:bool[])
            n182 = Reshape Array(w569, 2 ("dimension size"), 8 ("dimension size")) -> (w566:bool[][])
            n183 = for {
              tunnel: w566 -> [w575] mode=indexing
              tunnel: [w573] -> w557 mode=indexing
              n184 = Boolean Array To Number(Boolean array=w575) -> (number=w574:u32)
              n185 = To Unsigned Byte Integer(number=w574) -> (unsigned 8bit integer=w573:u8)
            }
            n186 = Initialize Array(u8 0, 128 ("dimension size")) -> (w531:u8[])
            n187 = Build Array (concatenate)(u8[] [53, 187, 37, 71, 79, 49, 4, 63] ("Array 2"), w557, w557) -> (w562:u8[])
            n188 = call "tx_pduGen.vi"("byte array"=w562) -> ("packet bits length"=→"packet bits length":i32, "pdu"=w533:i32[])  [unwired: 3 in]
            n189 = Build Array (concatenate)(w533, w532, w531) -> (w530:i32[])
            n190 = call "sub_bits_to_symbols.vi"("symbol map"=w547, "bits"=w530) -> ("symbols"=w546:cdb[])  [unwired: 9 in]
            n191 = Build Array (concatenate)(w546, w548) -> (w544:cdb[])
            n192 = call-poly <vilib>:"MT Pulse Shaping Filter.vi"("symbols"=w544, "pulse shaping filter coefficients"=w559, "samples per symbol (16)"=w554, "symbol rate (Hz)"=w558, "reset? (T)"=FALSE) -> ("output complex waveform"=w553:T9)  [unwired: 9 in, 1 out]
            n193 = Divide(x="Transmit power (db)", y=20.0) -> (x/y=w541:dbl)
            n194 = Unbundle(w553) -> ("t0"=w552:dbl, "dt"=w551:dbl, "Y"=w539:cdb[])
            n195 = Power Of 10(x=w541) -> (10^x=w540:dbl)
            n196 = Multiply(x=w539, y=w540) -> (x*y=w538:cdb[])
            n197 = Bundle(cluster=w553, "t0"=w552, "dt"=w551, "Y"=w538) -> (w550:T9)
            n198 = Enqueue Element(queue=w565, element=w550, error in (no error)=w563) -> (error out=w564:errorcluster)  [unwired: 1 in, 2 out]
          }
        }
        n199 = global read "var_stop.vi" "system stop"() -> (w517:bool)
      }
    }
    frame Error {
    }
  }
